vi "HostControl_Main_old.vi"() -> ()   [LabVIEW 2012]
uses:
  <vilib>/MakerHub/KinectOne/KinectOne.lvlib
  <vilib>/MakerHub/KinectOne/Private/Initialize Image [Color].vi
  Messages.ctl
  Support VIs/setpointCluster.ctl
  GainsTDef.ctl
  <vilib>/MakerHub/KinectOne/Private/kinectRead [ColorFrame].vi
  Support VIs/speeds.ctl
  PolarCoordTdef.ctl
  Support VIs/messageTypes.ctl
  Support VIs/operationModes.ctl
  StopTDef.ctl
  <vilib>/MakerHub/PS4-Controller/LMH-PS4.lvlib
  <vilib>/MakerHub/KinectOne/Private/kinectRead [BodyFrame].vi
  <vilib>/MakerHub/PS4-Controller/Public/Open First Controller.vi
  <vilib>/MakerHub/KinectOne/Private/Type Defs/ClippedEdges.ctl
  <vilib>/MakerHub/KinectOne/Private/Type Defs/HandLeftConfidence.ctl
  <vilib>/MakerHub/KinectOne/Private/Type Defs/HandLeftState.ctl
  <vilib>/MakerHub/KinectOne/Private/Type Defs/HandRightConfidence.ctl
  <vilib>/MakerHub/KinectOne/Private/Type Defs/HandRightState.ctl
  <vilib>/MakerHub/KinectOne/Private/Type Defs/LeanTrackingState.ctl
  <vilib>/MakerHub/KinectOne/Private/Type Defs/BodyData.ctl
  Microsoft.Kinect
panel:
  out "error out":errorcluster
  in  "colour mode (T = dist, F = sphere)":bool
  out "Detected Colour":u32(colorbox)
  out "Tracked?":bool
  in  "Forward Speed Limit [rad/s] (10 r/s)":dbl(knob)=2.995028509599303 scale=0.0..10.0
  out "Gains Closed":bool
  out "Setpoint\nGen Closed":bool
  out "Stopper\nClosed":bool
  out "Kinect Closed":bool
  out "Ctrl Event\nLoop Off":bool
  out "Controller Off":bool
  out "Hand Ctrl Closed":bool
  out "Message Sender Closed":bool
  in  "ControllerStop":bool
  out "Controller?":bool
  out "Toggle":bool
  in  "Cancel\nButton":bool
  out "TX":bool
  in  "bodyData":T1[](array[typedef])
  in  "Modulus SP":dbl=1.7999999523162842
  in  "Reference\nColour":u32(colorbox)
  in  "Argument SP":dbl
  out "index":i32
  in  "Operation Mode":T8 items=["TeleOp", "Desperate", "ColourMatch"]
  out "Image":T9(plugin-control)
  in  "Kd-Argument":dbl
  in  "Kc-Argument":dbl=0.30000001192092896
  in  "Kd-Modulus":dbl
  in  "Kc-Modulus":dbl=0.5
  out "Mod":dbl
  out "Arg":dbl
  in  "IT'S TIME TO":bool
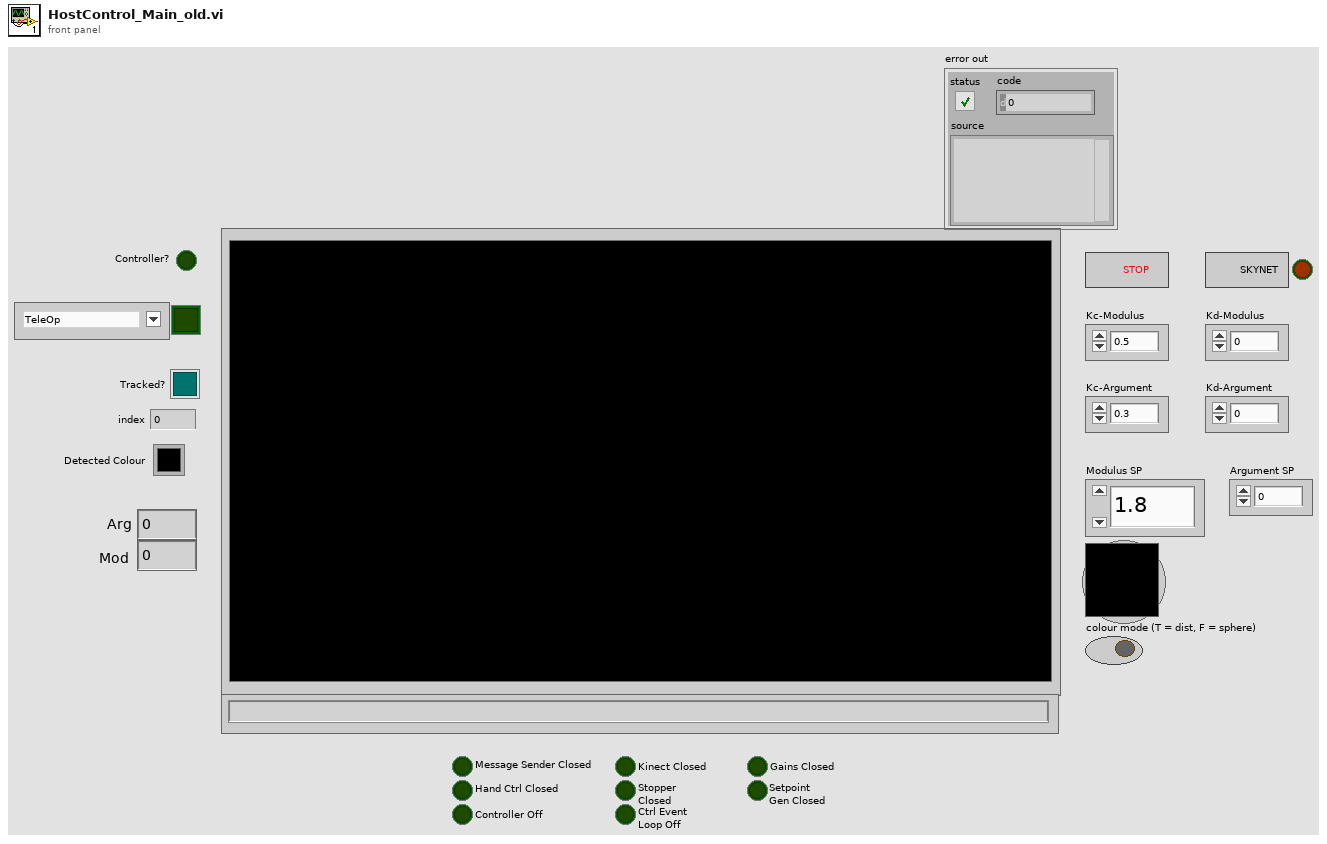
[diagram p1: front panel]
types:
  T1 = typedef "KinectOne.lvlib/BodyData.ctl" = cluster{"ClippedEdges":T2, "HandLeftConfidence":T3, "HandLeftState":T4, "HandRightConfidence":T5, "HandRightState":T6, "IsRestricted":bool, "IsTracked":bool, "JointOrientations":refnum<k24>, "Joints":refnum<k24>, "Lean":refnum<k24>, "LeanTrackingState":T7, "TrackingId":u64}
  T2 = typedef "KinectOne.lvlib/ClippedEdges.ctl" = enum16{"None", "Right", "Left", "Top", "Bottom"}
  T3 = typedef "KinectOne.lvlib/HandLeftConfidence.ctl" = enum16{"Low", "High"}
  T4 = typedef "KinectOne.lvlib/HandLeftState.ctl" = enum16{"Unknown", "NotTracked", "Open", "Closed", "Lasso"}
  T5 = typedef "KinectOne.lvlib/HandRightConfidence.ctl" = enum16{"Low", "High"}
  T6 = typedef "KinectOne.lvlib/HandRightState.ctl" = enum16{"Unknown", "NotTracked", "Open", "Closed", "Lasso"}
  T7 = typedef "KinectOne.lvlib/LeanTrackingState.ctl" = enum16{"NotTracked", "Inferred", "Tracked"}
  T8 = typedef "operationModes.ctl" = u16
  T9 = typedef "IMAQ Image.ctl" = refnum<image>
  T10 = typedef "GainsTDef.ctl" = cluster{"Kc-Modulus":sgl, "Kd-Modulus":sgl, "Kc-Argument":sgl, "Kd-Argument":sgl}
  T11 = typedef "Messages.ctl" = cluster{"message data":variant, "message type":T12}
  T12 = typedef "messageTypes.ctl" = enum16{"Speeds", "Stop", "PolarCoordinates", "Gains", "Setpoints"}
  T13 = typedef "StopTDef.ctl" = cluster{"stop":bool}
  T14 = typedef "KinectOne.lvlib/KinectSensor References.ctl" = cluster{"KinectSensor":refnum<k24>, "MultiSourceFrameReader":refnum<k24>, "BodyFrameDataInterface":refnum<k24>}
  T15 = typedef "LMH-PS4.lvlib/PS4 Controller Ref.ctl" = cluster{"Controller Ref":refnum<k1>, "PS4 Events Ref":refnum<event-registration>, "Worker Ref":refnum<vi>}
  T16 = typedef "setpointCluster.ctl" = cluster{"Modulus Setpoint":sgl, "Argument Setpoint":sgl}
  T17 = typedef "speeds.ctl" = cluster{"left motor [rad/s]":dbl, "right motor [rad/s]":dbl}
  T18 = typedef "PolarCoordTdef.ctl" = cluster{"Argument":dbl, "Modulus":dbl, "trackedState":bool}
  T19 = typedef "KinectOne.lvlib/Joint Position.ctl" = cluster{"Camera Space":cluster{"X":dbl, "Y":dbl, "Z":dbl}, "Color Space":cluster{"X":dbl, "Y":dbl}, "Depth Space":cluster{"X":dbl, "Y":dbl}, "Tracking State":enum16{"NotTracked", "Inferred", "Tracked"}}
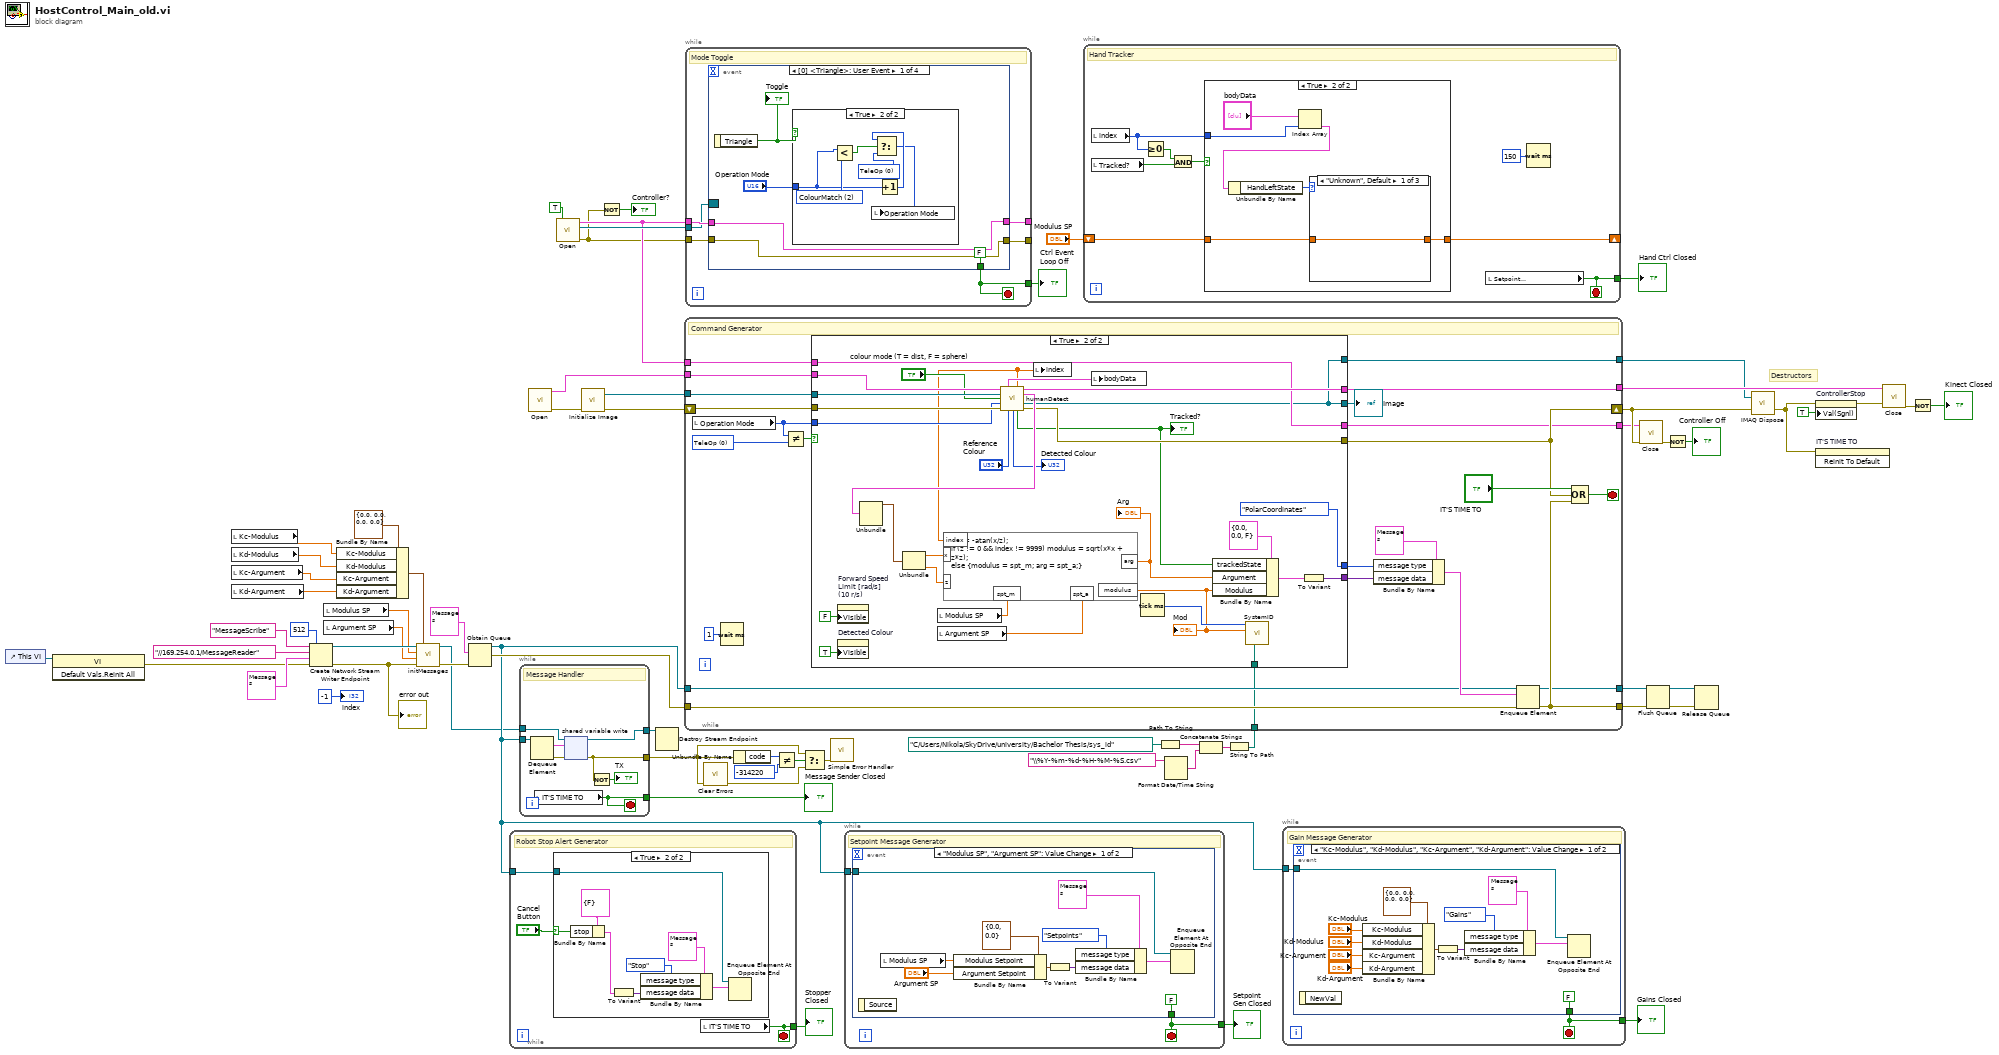
[diagram p0: block diagram]
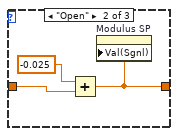
[diagram p3: hidden frame]
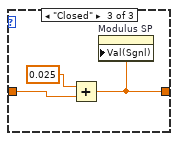
[diagram p4: hidden frame]
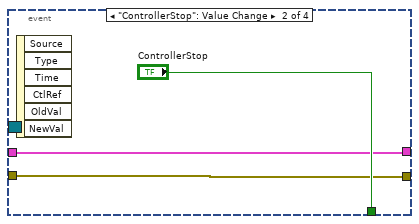
[diagram p6: hidden frame]
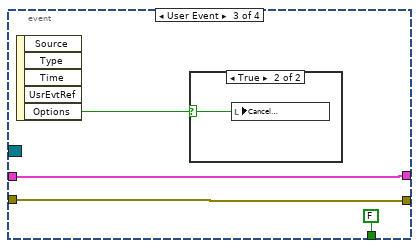
[diagram p7: hidden frame]
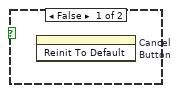
[diagram p8: hidden frame]
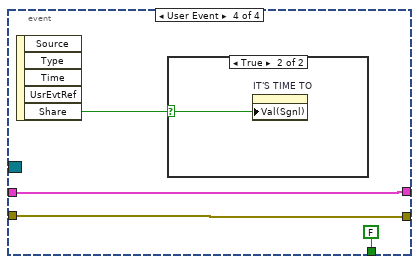
[diagram p9: hidden frame]
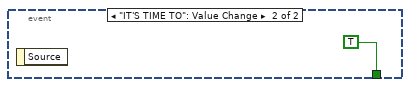
[diagram p12: hidden frame]
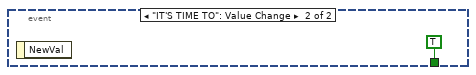
[diagram p13: hidden frame]
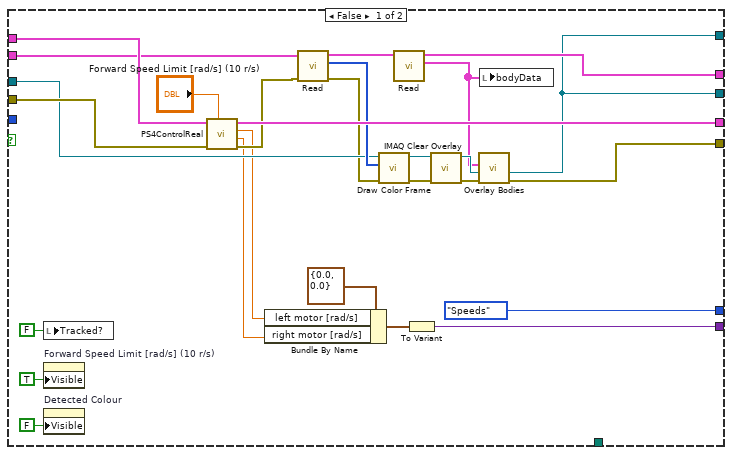
[diagram p14: hidden frame]
diagram:
  # "Destructors"
  n1 = control-ref of="This VI"() -> (w12:refnum<vi>)
  n2 = invoke class="VI" method="Default Vals.Reinit All"(reference=w12) -> (error out=w7:errorcluster)  [unwired: 2 in, 2 out]
  n3 = local read "Kc-Modulus"() -> (w37:dbl)
  n4 = local read "Kd-Modulus"() -> (w36:dbl)
  n5 = local read "Kc-Argument"() -> (w35:dbl)
  n6 = local read "Kd-Argument"() -> (w34:dbl)
  n7 = Create Network Stream Writer Endpoint(7:512 ("writer buffer size"), 8:w7, 9:T11 {"message data"=variant, "message type"=enum."Setpoints"} ("message"), 10:"//169.254.0.1/MessageReader" ("reader url"), 11:"MessageScribe" ("writer name")) -> (0:w8:errorcluster, 3:w32:refnum<k21>)  [unwired: 2 in]
  "error out" <- w8
  n8 = local read "Modulus SP"() -> (w31:dbl)
  n9 = local read "Argument SP"() -> (w30:dbl)
  n10 = Bundle By Name(cluster=T10 {"Kc-Modulus"=0.0, "Kd-Modulus"=0.0, "Kc-Argument"=0.0, "Kd-Argument"=0.0}, "Kc-Modulus"=w37, "Kd-Modulus"=w36, "Kc-Argument"=w35, "Kd-Argument"=w34) -> (w33:T10)
  n11 = call "initMessages.vi"("GainsCluster"=w33, "error in (no error)"=w8, "Argument Setpoint"=w30, "Modulus Setpoint"=w31, "writer name in"=w32) -> ("error out"=w29:errorcluster, "Refnum out"=w28:refnum<k21>)  [unwired: 5 in]
  n12 = Obtain Queue(element data type=T11 {"message data"=variant, "message type"=enum."Stop"} ("message"), error in (no error)=w29) -> (queue out=w55:refnum<queue>, error out=w62:errorcluster)  [unwired: 3 in, 1 out]
  n13 = while {
    tunnel: w55 -> [w69]
    tunnel: [w67] -> w15
    stop <- w67 stop-if-true
    # "Robot Stop Alert Generator"
    n14 = case shown="True" "Cancel\nButton" {
      selector: "Cancel\nButton" -> [_ w72]
      tunnel: w69 -> [_ w73]
      frame False {
      }
      frame True {
        n15 = Bundle By Name(cluster=T13 {"stop"=FALSE} ("Cluster"), "stop"=w72) -> (w70:T13)
        n16 = To Variant(anything=w70) -> (Variant=w76:variant)
        n17 = Bundle By Name(cluster=T11 {"message data"=variant, "message type"=enum."Stop"} ("message"), "message type"=messageTypes."Stop", "message data"=w76) -> (w75:T11)
        n18 = Enqueue Element At Opposite End(queue=w73, element=w75) -> ()  [unwired: 2 in, 3 out]
      }
    }
    n19 = local read "IT'S TIME TO"() -> (w67:bool)
  }
  "Stopper\nClosed" <- w15
  n20 = while {
    tunnel: w55 -> [w85]
    tunnel: [w83] -> w40
    tunnel: [w82] -> w39
    tunnel: w28 -> [w80]
    tunnel: [w79] -> w16
    stop <- w79 stop-if-true
    # "Message Handler"
    n21 = Dequeue Element(queue=w85) -> (element=w84:T11, error out=w78:errorcluster)  [unwired: 2 in, 2 out]
    n22 = local read "IT'S TIME TO"() -> (w79:bool)
    n23 = shared-variable-write(w80, w78, w84) -> (w83:refnum<k21>, w82:errorcluster)  [unwired: 1 in, 1 out]
    n24 = Not(x=w82) -> (.not. x?=→"TX":bool)
  }
  "Message Sender Closed" <- w16
  n25 = call <vilib>:"Open.vi"() -> ("Error Out"=w66:errorcluster, "KinectSensor References out"=w58:T14)  [unwired: 10 in]
  n26 = call-poly <vilib>:"Open.vi"("Enable Events (T)"=TRUE) -> ("Error Out"=w27:errorcluster, "Event Registration Refnum"=w59:refnum<event-registration>, "PS4 Controller Ref"=w57:T15)  [unwired: 8 in]
  n27 = call-poly <vilib>:"Initialize Image.vi"("Error In"=w66) -> ("Error Out"=w65:errorcluster, "Color Image"=w64:T9)  [unwired: 9 in]
  n28 = Not(x=w27) -> (.not. x?=→"Controller?":bool)
  n29 = Destroy Stream Endpoint(11:w40) -> ()  [unwired: 1 in, 1 out]
  n30 = while {
    tunnel: w59 -> [w89]
    tunnel: w27 -> [w90]
    tunnel: [w87] -> _
    tunnel: w57 -> [w91]
    tunnel: [w88] -> _
    tunnel: [w86] -> w17
    stop <- w86 stop-if-true
    # "Mode Toggle"
    n31 = event shown="[0] <Triangle>: User Event" {
      selector: w89 -> [_ _ _ _]
      dyn-events: _ -> [_ _ _ _]
      timeout: _ -> [_ _ _ _]
      tunnel: w91 -> [w94 w104 w108 w113]
      tunnel: w90 -> [w93 w103 w107 w112]
      tunnel: [w94 w104 w108 w113] -> w88
      tunnel: [w93 w103 w107 w112] -> w87
      tunnel: [FALSE ("ControllerStop") "ControllerStop" FALSE ("ControllerStop") FALSE ("ControllerStop")] -> w86
      event User Event {
        n32 = event-data() -> ("Triangle"=w96:bool)  [unwired: 1 in]
        "Toggle" <- w96
        n33 = case shown="True" w96 {
          tunnel: "Operation Mode" -> [_ w97]
          frame False {
          }
          frame True {
            w98 = T8 2 items=["TeleOp", "Desperate", "ColourMatch"] ("Operation Mode 2")
            w99 = T8 0 items=["TeleOp", "Desperate", "ColourMatch"] ("Operation Mode 2")
            n34 = Less?(x=w97, y=w98) -> (x < y?=w102:bool)
            n35 = Increment(x=w97) -> (x+1=w101:T8)
            n36 = Select(t=w101, s=w102, f=w99) -> (s? t:f=w100:T8)
            n37 = local write "Operation Mode"(w100) -> ()
          }
        }
      }
      event "ControllerStop": Value Change {
        n38 = event-data() -> ()  [unwired: 1 in, 6 out]
      }
      event User Event {
        n39 = event-data() -> ("Options"=w109:bool)  [unwired: 1 in, 4 out]
        n40 = case shown="True" w109 {
          selector: w109 -> [_ w110]
          frame False {
            n41 = invoke on="Cancel\nButton" class="Bool (strict)" method="Reinit To Default"() -> ()  [unwired: 3 in, 3 out]
          }
          frame True {
            n42 = local write "Cancel\nButton"(w110) -> ()
          }
        }
      }
      event User Event {
        n43 = event-data() -> ("Share"=w114:bool)  [unwired: 1 in, 4 out]
        n44 = case shown="True" w114 {
          selector: w114 -> [_ w115]
          frame False {
          }
          frame True {
            n45 = property on="IT'S TIME TO" class="Bool (strict)"("Val(Sgnl)"=w115) -> ()  [unwired: 2 in, 2 out]
          }
        }
      }
    }
  }
  "Ctrl Event\nLoop Off" <- w17
  n46 = call <vilib>:"Clear Errors.vi"("error in (no error)"=w39) -> ("error out"=w47:errorcluster)  [unwired: 6 in]
  n47 = Unbundle By Name(w39) -> ("code"=w48:i32)
  n48 = Not Equal?(x=w48, y=-314220) -> (x != y?=w50:bool)
  n49 = Select(t=w39, s=w50, f=w47) -> (s? t:f=w41:errorcluster)
  n50 = call <vilib>:"Simple Error Handler.vi"("error in (no error)"=w41) -> ()  [unwired: 4 in, 5 out]
  n51 = while {
    tunnel: w55 -> [w117]
    tunnel: [w116] -> w13
    stop <- w116 stop-if-true
    # "Setpoint Message Generator"
    n52 = event shown="[0] \"Modulus SP\", \"Argument SP\": Value Change" {
      selector: _ -> [_ _]
      dyn-events: _ -> [_ _]
      timeout: _ -> [_ _]
      tunnel: w117 -> [w123 _]
      tunnel: [FALSE TRUE] -> w116
      event "Modulus SP", "Argument SP": Value Change {
        n53 = event-data() -> ()  [unwired: 1 in, 1 out]
        n54 = local read "Modulus SP"() -> (w121:dbl)
        n55 = Bundle By Name(cluster=T16 {"Modulus Setpoint"=0.0, "Argument Setpoint"=0.0} ("Setpoint Cluster"), "Modulus Setpoint"=w121, "Argument Setpoint"="Argument SP") -> (w122:T16)
        n56 = To Variant(anything=w122) -> (Variant=w125:variant)
        n57 = Bundle By Name(cluster=T11 {"message data"=variant, "message type"=enum."Stop"} ("message"), "message type"=messageTypes."Setpoints", "message data"=w125) -> (w124:T11)
        n58 = Enqueue Element At Opposite End(queue=w123, element=w124) -> ()  [unwired: 2 in, 3 out]
      }
      event "IT'S TIME TO": Value Change {
        n59 = event-data() -> ()  [unwired: 1 in, 1 out]
      }
    }
  }
  "Setpoint\nGen Closed" <- w13
  n60 = while {
    shift-right: [w130] -> _
    shift-left: "Modulus SP" -> [w132]
    tunnel: [w129] -> w10
    stop <- w129 stop-if-true
    # "Hand Tracker"
    n61 = local read "index"() -> (w133:i32)
    n62 = local read "Tracked?"() -> (w134:bool)
    n63 = Greater Or Equal To 0?(x=w133) -> (x >= 0?=w135:bool)
    n64 = And(x=w135, y=w134) -> (x .and. y?=w136:bool)
    n65 = case shown="True" w136 {
      tunnel: w133 -> [_ w143]
      tunnel: w132 -> [w137 w140]
      tunnel: [w137 w138] -> w130
      frame False {
      }
      frame True {
        n66 = Index Array(array="bodyData", index=w143) -> (element=w142:T1)
        n67 = Unbundle By Name(w142) -> ("HandLeftState"=w141:T4)
        n68 = case shown="\"Unknown\", Default" w141 {
          tunnel: w140 -> [w144 w146 w149]
          tunnel: [w144 w145 w148] -> w138
          frame "Unknown", Default {
          }
          frame "Open" {
            n69 = Add(x=-0.025, y=w146) -> (x+y=w145:dbl)
            n70 = property on="Modulus SP" class="DigNum (strict)"("Val(Sgnl)"=w145) -> ()  [unwired: 2 in, 2 out]
          }
          frame "Closed" {
            n71 = Add(x=0.025, y=w149) -> (x+y=w148:dbl)
            n72 = property on="Modulus SP" class="DigNum (strict)"("Val(Sgnl)"=w148) -> ()  [unwired: 2 in, 2 out]
          }
        }
      }
    }
    n73 = local read "Setpoint\nGen Closed"() -> (w129:bool)
    n74 = Wait (ms)(milliseconds to wait=u32 150) -> ()  [unwired: 1 out]
  }
  "Hand Ctrl Closed" <- w10
  n75 = Path To String(path=path "C:/Users/Nikola/SkyDrive/university/Bachelor Thesis/sys_id" ("file path (dialog if empty)")) -> (string=w4:string)
  n76 = Format Date/Time String(time format string (%c)="\\%Y-%m-%d-%H-%M-%S.csv") -> (date/time string=w2:string)  [unwired: 2 in]
  n77 = Concatenate Strings(w4, w2) -> (w3:string)
  n78 = String To Path(string=w3) -> (path=w1:path)
  n79 = while {
    tunnel: w58 -> [w168]
    tunnel: w64 -> [w167]
    shift-right: [w166] -> w22
    shift-left: w65 -> [w165]
    tunnel: [w163] -> w63
    tunnel: w55 -> [w169]
    tunnel: [w164] -> w60
    tunnel: [w154] -> w52
    tunnel: w57 -> [w161]
    tunnel: [w160] -> w21
    tunnel: w62 -> [w171]
    tunnel: [w170] -> w51
    tunnel: w1 -> [w151]
    stop <- w174 stop-if-true
    w156 = T8 0 items=["TeleOp", "Desperate", "ColourMatch"] ("y")
    # "Command Generator"
    n80 = local read "Operation Mode"() -> (w157:T8)
    n81 = Wait (ms)(milliseconds to wait=u32 1) -> ()  [unwired: 1 out]
    n82 = Not Equal?(x=w157, y=w156) -> (x != y?=w162:bool)
    n83 = case shown="True" w162 {
      tunnel: w168 -> [w198 w229]
      tunnel: w167 -> [w196 w228]
      tunnel: [w177 w226] -> w166
      tunnel: w165 -> [w200 w225]
      tunnel: [w178 w215] -> w164
      tunnel: [w181 w224] -> w163
      tunnel: w161 -> [w201 w217]
      tunnel: [w199 w217] -> w160
      tunnel: w157 -> [_ w221]
      tunnel: [messageTypes."Speeds" ("message type") messageTypes."PolarCoordinates" ("message type")] -> w159
      tunnel: [w189 w219] -> w158
      tunnel: [w178 w215] -> w153
      tunnel: w151 -> [_ w207]
      frame False {
        n84 = local write "Tracked?"(FALSE) -> ()
        n85 = property on="Forward Speed Limit [rad/s] (10 r/s)" class="Knob (strict)"("Visible"=TRUE) -> ()  [unwired: 2 in, 2 out]
        n86 = property on="Detected Colour" class="ColBox"("Visible"=FALSE) -> ()  [unwired: 2 in, 2 out]
        n87 = call "PS4ControlReal.vi"("Forward Speed Limit [rad/s] (10.7 r/s)"="Forward Speed Limit [rad/s] (10 r/s)", "Error In"=w200, "PS4 Controller Ref In"=w201) -> ("Error Out"=w195:errorcluster, "right motor out"=w192:dbl, "left motor out"=w193:dbl, "PS4 Controller Ref Out"=w199:T15)  [unwired: 5 in]
        n88 = Bundle By Name(cluster=T17 {"left motor [rad/s]"=0.0, "right motor [rad/s]"=0.0}, "left motor [rad/s]"=w193, "right motor [rad/s]"=w192) -> (w190:T17)
        n89 = call-poly <vilib>:"Read.vi"("Error In"=w195, "KinectSensor References in"=w198) -> ("Error Out"=w194:errorcluster, "frameData"=w197:u32[], "KinectSensor References out"=w182:T14)  [unwired: 7 in]
        n90 = call <vilib>:"Draw Color Frame.vi"("Error In"=w194, "U32 Array"=w197, "Image"=w196) -> ("Error Out"=w180:errorcluster, "Image Out"=w184:T9)  [unwired: 7 in]
        n91 = call-poly <vilib>:"Read.vi"("KinectSensor References in"=w182) -> ("Body Data"=w176:T1[], "KinectSensor References out"=w181:T14)  [unwired: 8 in, 1 out]
        n92 = To Variant(anything=w190) -> (Variant=w189:variant)
        n93 = call "IMAQ Clear Overlay"("error in (no error)"=w180, "Image"=w184) -> ("error out"=w179:errorcluster, "Image Out"=w183:T9)  [unwired: 8 in]
        n94 = call <vilib>:"Overlay Bodies.vi"("Error In"=w179, "Image"=w183, "Body Data"=w176) -> ("Error Out"=w177:errorcluster, "Image Out"=w178:T9)  [unwired: 7 in]
        n95 = local write "bodyData"(w176) -> ()
      }
      frame True {
        n96 = property on="Forward Speed\nLimit [rad/s] \n(10 r/s)" class="Knob (strict)"("Visible"=FALSE) -> ()  [unwired: 2 in, 2 out]
        n97 = property on="Detected Colour" class="ColBox"("Visible"=TRUE) -> ()  [unwired: 2 in, 2 out]
        n98 = local read "Modulus SP"() -> (w208:dbl)
        n99 = local read "Argument SP"() -> (w223:dbl)
        n100 = call "humanDetect.vi"("KinectSensor References in"=w229, "Tracker"=w228, "colour mode (T = dist, F = sphere)"="colour mode (T = dist, F = sphere)", "Operation Mode"=w221, "Error In"=w225, "Reference Colour"="Reference\nColour") -> ("Body Data"=w216:T1[], "index"=w209:sgl, "KinectSensor References"=w224:T14, "Joint Position"=w227:T19, "Image"=w215:T9, "Averaged Colour"=→"Detected Colour":u32, "istracked"=w213:bool, "Error Out"=w226:errorcluster)  [unwired: 2 in]
        "Tracked?" <- w213
        n101 = Unbundle(w227) -> ("Camera Space"=w231:cluster{"X":dbl, "Y":dbl, "Z":dbl})  [unwired: 3 out]
        n102 = Unbundle(w231) -> ("X"=w203:dbl, "Z"=w202:dbl)  [unwired: 1 out]
        n103 = formula code="arg = -atan(x/z);\nif (z != 0 && index != 9999) modulus = sqrt(x*x + z*z);\nelse {modulus = spt_m; arg = spt_a;}"("x"=w203, "z"=w202, "spt_m"=w208, "spt_a"=w223, "index"=w209) -> ("arg"=w205:dbl, "modulus"=w204:dbl)
        "Arg" <- w205
        "Mod" <- w204
        n104 = local write "index"(w209) -> ()
        n105 = local write "bodyData"(w216) -> ()
        n106 = Tick Count (ms)() -> (millisecond timer value=w206:u32)
        n107 = Bundle By Name(cluster=T18 {"Argument"=0.0, "Modulus"=0.0, "trackedState"=FALSE}, "trackedState"=w213, "Argument"=w205, "Modulus"=w204) -> (w220:T18)
        n108 = call "SystemID.vi"("file path (dialog if empty)"=w207, "Value"=w204, "Time"=w206) -> ()  [unwired: 8 in, 1 out]
        n109 = To Variant(anything=w220) -> (Variant=w219:variant)
      }
    }
    "Image" <- w153
    n110 = Bundle By Name(cluster=T11 {"message data"=variant, "message type"=enum."Stop"} ("message"), "message type"=w159, "message data"=w158) -> (w172:T11)
    n111 = Enqueue Element(queue=w169, element=w172, error in (no error)=w171) -> (queue out=w154:refnum<queue>, error out=w170:errorcluster)  [unwired: 1 in, 1 out]
    n112 = Compound Arithmetic op=OR("IT'S TIME TO", w166, w170) -> (w174:bool)
  }
  n113 = while {
    tunnel: w55 -> [w233]
    tunnel: [w232] -> w14
    stop <- w232 stop-if-true
    # "Gain Message Generator"
    n114 = event shown="[0] \"Kc-Modulus\", \"Kd-Modulus\", \"Kc-Argument\", \"Kd-Argument\": Value Change" {
      selector: _ -> [_ _]
      dyn-events: _ -> [_ _]
      timeout: _ -> [_ _]
      tunnel: w233 -> [w236 _]
      tunnel: [FALSE TRUE] -> w232
      event "Kc-Modulus", "Kd-Modulus", "Kc-Argument", "Kd-Argument": Value Change {
        n115 = event-data() -> ()  [unwired: 1 in, 1 out]
        n116 = Bundle By Name(cluster=T10 {"Kc-Modulus"=0.0, "Kd-Modulus"=0.0, "Kc-Argument"=0.0, "Kd-Argument"=0.0}, "Kc-Modulus"="Kc-Modulus", "Kd-Modulus"="Kd-Modulus", "Kc-Argument"="Kc-Argument", "Kd-Argument"="Kd-Argument") -> (w240:T10)
        n117 = To Variant(anything=w240) -> (Variant=w239:variant)
        n118 = Bundle By Name(cluster=T11 {"message data"=variant, "message type"=enum."Stop"} ("message"), "message type"=messageTypes."Gains", "message data"=w239) -> (w237:T11)
        n119 = Enqueue Element At Opposite End(queue=w236, element=w237) -> ()  [unwired: 2 in, 3 out]
      }
      event "IT'S TIME TO": Value Change {
        n120 = event-data() -> ()  [unwired: 1 in, 1 out]
      }
    }
  }
  "Gains Closed" <- w14
  n121 = call <vilib>:"Close.vi"("Error In"=w22, "PS4 Controller Ref"=w21) -> ("Error Out"=w9:errorcluster)  [unwired: 9 in]
  n122 = Flush Queue(queue=w52, error in (no error)=w51) -> (queue out=w54:refnum<queue>, error out=w53:errorcluster)  [unwired: 1 out]
  n123 = Not(x=w9) -> (.not. x?=→"Controller Off":bool)
  n124 = Release Queue(queue=w54, error in (no error)=w53) -> ()  [unwired: 1 in, 3 out]
  n125 = call "IMAQ Dispose"("Image"=w60, "error in (no error)"=w22) -> ("error out"=w11:errorcluster)  [unwired: 4 in]
  n126 = property on="ControllerStop" class="Bool (strict)"(error in=w11, "Val(Sgnl)"=TRUE ("Value (Signaling)")) -> (error out=w24:errorcluster)  [unwired: 1 in, 1 out]
  n127 = invoke on="IT'S TIME TO" class="Bool (strict)" method="Reinit To Default"(error in=w11) -> ()  [unwired: 2 in, 3 out]
  n128 = call <vilib>:"Close.vi"("Error In"=w24, "KinectSensor References"=w63) -> ("Error Out"=w19:errorcluster)  [unwired: 9 in]
  n129 = Not(x=w19) -> (.not. x?=→"Kinect Closed":bool)
  "index" <- -1 ("index")
